vi "H5_ReadAttr.vi"(0 "HDF5 Ref In":T1, 7 "error in (no error)":errorcluster) -> (1 "X Start":sgl, 2 "X End":sgl=10.0, 3 "Y Start":sgl, 4 "Y End":sgl=8.0, 5 "Scan Mode":enum16{"Raster", "Serpentine"}(ring), 6 "Speed Control (mm/s)":sgl=1.0 min=0.1, 8 "Scan Time (Approx.)":string, 9 "Pixel Count":i32=6 caption="X Pixels", 10 "X Step Size (R)":sgl format="%#_2g", 11 "Line Count":i32=6 caption="Y Pixels", 12 "Y Step Size (R)":sgl format="%#_2g", 13 "Gen Sampling Rate":u64, 14 "Amplitudes (V)":sgl[](array[numeric]) format="%#_2g", 15 "Contact Info":string, 16 "Offset":sgl format="%#_2g", 17 "Gain":sgl format="%#_2g", 18 "Waves per Pixel":u16, 19 "Record Size":u16=1024, 20 "HDF5 Ref Out":T1, 21 "Delay(us)":sgl min=0 step=0.1 format="%#_4g", 22 "Sampling Freq (Hz)":sgl min=0 step=0.1 format="%#_4g", 23 "Temperature":sgl min=0 step=0.1 format="%#_4g", 24 "Remarks":string="Notes: Scanned in UiT", 25 "Transducer Freq(Hz)":u64 step=1, 26 "Immersion Medium":string="Water", 27 "error out":errorcluster)   [LabVIEW 2020]
uses:
  <vilib>/UPVI/lvhdf5/library.llb/HDF5 Ref.ctl
  <vilib>/UPVI/lvhdf5/group.llb/OpenCreateGroup (String).vi
  <vilib>/UPVI/lvhdf5/attribute.llb/Simple H5Aread (Variant).vi
  <vilib>/UPVI/lvhdf5/attribute.llb/Simple H5Aread.xnode
  <vilib>/UPVI/lvhdf5/attribute.llb/LVH5A Operation.ctl
  <vilib>/UPVI/lvhdf5/attribute.llb/LVH5 Write Attributes.xnode
  <vilib>/Utility/VariantDataType/GetClusterInfo.vi
  <vilib>/Utility/VariantDataType/VariantType.lvlib
  <vilib>/Utility/VariantDataType/GetTypeInfo.vi
  <vilib>/UPVI/lvhdf5/attribute.llb/Cluster to Attribute Array.xnode
  <vilib>/UPVI/lvhdf5/attribute.llb/Write Multiple Attributes.vi
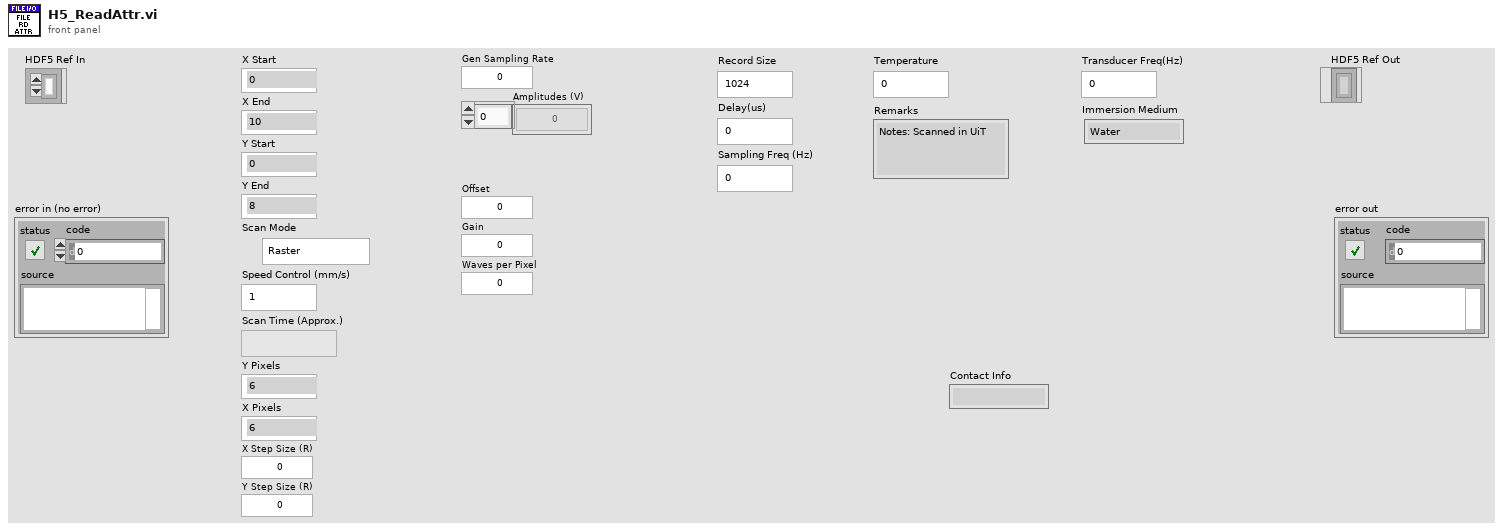
[diagram p1: front panel]
types:
  T1 = typedef "HDF5 Ref.ctl" = refnum<k1>
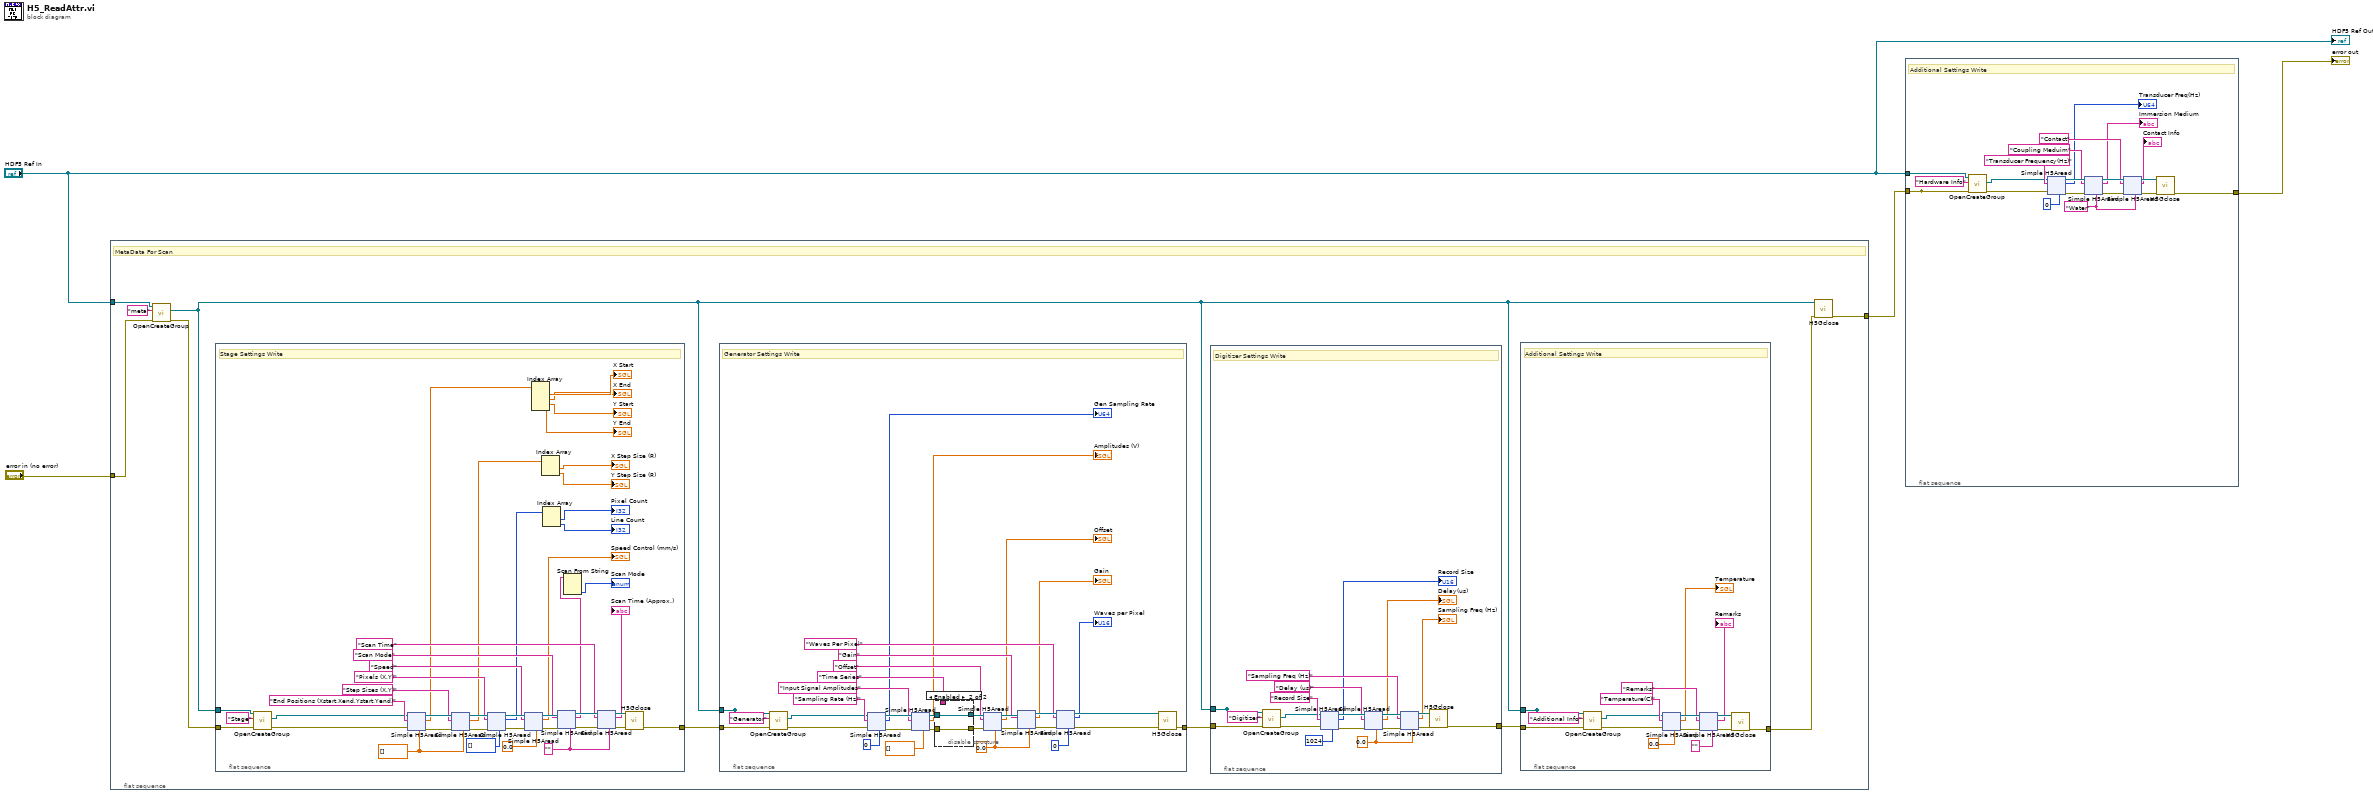
[diagram p0: block diagram]
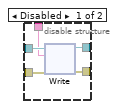
[diagram p2: hidden frame]
diagram:
  n1 = flat-sequence {
    tunnel: "error in (no error)" -> [w9]
    tunnel: "HDF5 Ref In" -> [w11]
    tunnel: [w5] -> w3
    frame #0 {
      # "MetaData For Scan"
      n2 = call-poly <vilib>:"OpenCreateGroup.vi"("error in (no error)"=w9, "Group"="meta", "HDF5 Ref"=w11) -> ("error out"=w10:errorcluster, "HDF5 Group Ref"=w7:T1)  [unwired: 6 in, 1 out]
      n3 = flat-sequence {
        tunnel: w10 -> [w478]
        tunnel: w7 -> [w477]
        tunnel: [w475] -> w14
        frame #0 {
          w472 = "" ("resulting string")
          w465 = sgl[] [] ("appended array")
          # "Stage Settings Write"
          n4 = call-poly <vilib>:"OpenCreateGroup.vi"("error in (no error)"=w478, "Group"="Stage", "HDF5 Ref"=w477) -> ("error out"=w481:errorcluster, "HDF5 Group Ref"=w480:T1)  [unwired: 6 in, 1 out]
          n5 = xnode "Simple H5Aread"("HDF5 Ref"=w480, "Name"="End Positions (Xstart,Xend,Ystart,Yend)", "error in (no error)"=w481, "Type"=w465) -> ("HDF5 Ref out"=w496:T1, "error out"=w495:errorcluster, "Value"=w471:sgl[])
          n6 = xnode "Simple H5Aread"("HDF5 Ref"=w496, "Name"="Step Sizes (X,Y)", "error in (no error)"=w495, "Type"=w465) -> ("HDF5 Ref out"=w494:T1, "error out"=w493:errorcluster, "Value"=w462:sgl[])
          n7 = xnode "Simple H5Aread"("HDF5 Ref"=w494, "Name"="Pixels (X,Y)", "error in (no error)"=w493, "Type"=i32[] [] ("appended array")) -> ("HDF5 Ref out"=w492:T1, "error out"=w491:errorcluster, "Value"=w459:i32[])
          n8 = xnode "Simple H5Aread"("HDF5 Ref"=w492, "Name"="Speed", "error in (no error)"=w491, "Type"=sgl 0.0 ("Speed Control (mm/s)")) -> ("HDF5 Ref out"=w490:T1, "error out"=w489:errorcluster, "Value"=→"Speed Control (mm/s)":sgl)
          n9 = Index Array(array=w471) -> (element #1=→"X Start":sgl, element #2=→"X End":sgl, element #3=→"Y Start":sgl, element #4=→"Y End":sgl)  [unwired: 4 in]
          n10 = Index Array(array=w462) -> (element #1=→"X Step Size (R)":sgl, element #2=→"Y Step Size (R)":sgl)  [unwired: 2 in]
          n11 = Index Array(array=w459) -> (element #1=→"Pixel Count":i32, element #2=→"Line Count":i32)  [unwired: 2 in]
          n12 = xnode "Simple H5Aread"("HDF5 Ref"=w490, "Name"="Scan Mode", "error in (no error)"=w489, "Type"=w472) -> ("HDF5 Ref out"=w488:T1, "error out"=w487:errorcluster, "Value"=w457:string)
          n13 = Scan From String(input string=w457) -> (output 1=→"Scan Mode":enum16{"Raster", "Serpentine"})  [unwired: 4 in, 3 out]
          n14 = xnode "Simple H5Aread"("HDF5 Ref"=w488, "Name"="Scan Time", "error in (no error)"=w487, "Type"=w472) -> ("HDF5 Ref out"=w474:T1, "error out"=w476:errorcluster, "Value"=→"Scan Time (Approx.)":string)
          n15 = call <vilib>:"H5Gclose.vi"("error in (no error)"=w476, "HDF5 Group Ref"=w474) -> ("error out"=w475:errorcluster)  [unwired: 7 in]
        }
      }
      n16 = flat-sequence {
        tunnel: w14 -> [w189]
        tunnel: [w185] -> _
        tunnel: [w187] -> w13
        tunnel: w7 -> [w185]
        frame #0 {
          w182 = sgl 0.0 ("Offset")
          # "Generator Settings Write"
          n17 = call-poly <vilib>:"OpenCreateGroup.vi"("error in (no error)"=w189, "Group"="Generator", "HDF5 Ref"=w185) -> ("error out"=w192:errorcluster, "HDF5 Group Ref"=w191:T1)  [unwired: 6 in, 1 out]
          n18 = xnode "Simple H5Aread"("HDF5 Ref"=w191, "Name"="Sampling Rate (Hz)", "error in (no error)"=w192, "Type"=u64 0 ("Gen Sampling Rate")) -> ("HDF5 Ref out"=w207:T1, "error out"=w206:errorcluster, "Value"=→"Gen Sampling Rate":u64)
          n19 = xnode "Simple H5Aread"("HDF5 Ref"=w207, "Name"="Input Signal Amplitudes", "error in (no error)"=w206, "Type"=sgl[] [] ("Amplitudes (V)")) -> ("HDF5 Ref out"=w205:T1, "error out"=w204:errorcluster, "Value"=→"Amplitudes (V)":sgl[])
          n20 = disable-structure shown="Enabled" {
            disable-tunnel: w205 -> [w338 w454]
            disable-tunnel: w204 -> [w337 w453]
            disable-tunnel: [w336 w454] -> w203
            disable-tunnel: [w335 w453] -> w202
            disable-tunnel: "Time Series" -> [w334 _]
            frame Disabled {
              n21 = xnode "Write"("HDF5 Ref"=w338, "error in (no error)"=w337, "Name(s)"=w334) -> ("HDF5 Ref out"=w336:T1, "error out"=w335:errorcluster)  [unwired: 2 in]
            }
            frame Enabled {
            }
          }
          n22 = xnode "Simple H5Aread"("HDF5 Ref"=w203, "Name"="Offset", "error in (no error)"=w202, "Type"=w182) -> ("HDF5 Ref out"=w201:T1, "error out"=w200:errorcluster, "Value"=→"Offset":sgl)
          n23 = xnode "Simple H5Aread"("HDF5 Ref"=w201, "Name"="Gain", "error in (no error)"=w200, "Type"=w182) -> ("HDF5 Ref out"=w199:T1, "error out"=w198:errorcluster, "Value"=→"Gain":sgl)
          n24 = xnode "Simple H5Aread"("HDF5 Ref"=w199, "Name"="Waves Per Pixel", "error in (no error)"=w198, "Type"=u16 0 ("Waves per Pixel")) -> ("HDF5 Ref out"=w186:T1, "error out"=w188:errorcluster, "Value"=→"Waves per Pixel":u16)
          n25 = call <vilib>:"H5Gclose.vi"("error in (no error)"=w188, "HDF5 Group Ref"=w186) -> ("error out"=w187:errorcluster)  [unwired: 7 in]
        }
      }
      n26 = flat-sequence {
        tunnel: w13 -> [w88]
        tunnel: w7 -> [w86]
        tunnel: [w87] -> w8
        tunnel: [w86] -> _
        frame #0 {
          w84 = sgl 0.0 ("Delay(us)")
          # "Digitizer Settings Write"
          n27 = call-poly <vilib>:"OpenCreateGroup.vi"("error in (no error)"=w88, "Group"="Digitizer", "HDF5 Ref"=w86) -> ("error out"=w91:errorcluster, "HDF5 Group Ref"=w90:T1)  [unwired: 6 in, 1 out]
          n28 = xnode "Simple H5Aread"("HDF5 Ref"=w90, "Name"="Record Size", "error in (no error)"=w91, "Type"=u16 1024 ("Record Size")) -> ("HDF5 Ref out"=w99:T1, "error out"=w98:errorcluster, "Value"=→"Record Size":u16)
          n29 = xnode "Simple H5Aread"("HDF5 Ref"=w99, "Name"="Delay (us)", "error in (no error)"=w98, "Type"=w84) -> ("HDF5 Ref out"=w97:T1, "error out"=w96:errorcluster, "Value"=→"Delay(us)":sgl)
          n30 = xnode "Simple H5Aread"("HDF5 Ref"=w97, "Name"="Sampling Freq (Hz)", "error in (no error)"=w96, "Type"=w84) -> ("HDF5 Ref out"=w95:T1, "error out"=w94:errorcluster, "Value"=→"Sampling Freq (Hz)":sgl)
          n31 = call <vilib>:"H5Gclose.vi"("error in (no error)"=w94, "HDF5 Group Ref"=w95) -> ("error out"=w87:errorcluster)  [unwired: 7 in]
        }
      }
      n32 = flat-sequence {
        tunnel: w8 -> [w21]
        tunnel: w7 -> [w19]
        tunnel: [w20] -> w6
        tunnel: [w19] -> _
        frame #0 {
          # "Additional Settings Write"
          n33 = call-poly <vilib>:"OpenCreateGroup.vi"("error in (no error)"=w21, "Group"="Additional Info", "HDF5 Ref"=w19) -> ("error out"=w24:errorcluster, "HDF5 Group Ref"=w23:T1)  [unwired: 6 in, 1 out]
          n34 = xnode "Simple H5Aread"("HDF5 Ref"=w23, "Name"="Temperature(C)", "error in (no error)"=w24, "Type"=sgl 0.0 ("Temperature")) -> ("HDF5 Ref out"=w29:T1, "error out"=w28:errorcluster, "Value"=→"Temperature":sgl)
          n35 = xnode "Simple H5Aread"("HDF5 Ref"=w29, "Name"="Remarks", "error in (no error)"=w28, "Type"="" ("Remarks")) -> ("HDF5 Ref out"=w27:T1, "error out"=w26:errorcluster, "Value"=→"Remarks":string)
          n36 = call <vilib>:"H5Gclose.vi"("error in (no error)"=w26, "HDF5 Group Ref"=w27) -> ("error out"=w20:errorcluster)  [unwired: 7 in]
        }
      }
      n37 = call <vilib>:"H5Gclose.vi"("error in (no error)"=w6, "HDF5 Group Ref"=w7) -> ("error out"=w5:errorcluster)  [unwired: 7 in]
    }
  }
  n38 = flat-sequence {
    tunnel: [w658] -> _
    tunnel: [w660] -> w1
    tunnel: "HDF5 Ref In" -> [w659]
    tunnel: w3 -> [w658]
    frame #0 {
      w651 = "Water" ("Immersion Medium")
      # "Additional Settings Write"
      n39 = call-poly <vilib>:"OpenCreateGroup.vi"("error in (no error)"=w658, "Group"="Hardware Info", "HDF5 Ref"=w659) -> ("error out"=w663:errorcluster, "HDF5 Group Ref"=w662:T1)  [unwired: 6 in, 1 out]
      n40 = xnode "Simple H5Aread"("HDF5 Ref"=w662, "Name"="Transducer Frequency(Hz)", "error in (no error)"=w663, "Type"=u64 0 ("Transducer Freq(Hz)")) -> ("HDF5 Ref out"=w666:T1, "error out"=w665:errorcluster, "Value"=→"Transducer Freq(Hz)":u64)
      n41 = xnode "Simple H5Aread"("HDF5 Ref"=w666, "Name"="Coupling Meduim", "error in (no error)"=w665, "Type"=w651) -> ("HDF5 Ref out"=w657:T1, "error out"=w656:errorcluster, "Value"=→"Immersion Medium":string)
      n42 = xnode "Simple H5Aread"("HDF5 Ref"=w657, "Name"="Contact", "error in (no error)"=w656, "Type"=w651) -> ("HDF5 Ref out"=w655:T1, "error out"=w654:errorcluster, "Value"=→"Contact Info":string)
      n43 = call <vilib>:"H5Gclose.vi"("error in (no error)"=w654, "HDF5 Group Ref"=w655) -> ("error out"=w660:errorcluster)  [unwired: 7 in]
    }
  }
  "error out" <- w1
  "HDF5 Ref Out" <- "HDF5 Ref In"
